vi "NextToken.vi"(7 "error in (no error)":errorcluster, 9 "Index In":i32, 10 "JSON String":string) -> (0 "error out":errorcluster, 1 "TOKEN":T1, 2 "Index Out":i32, 3 "JSON String Passthrough":string)   [LabVIEW 2010, in "i3-json.lvlib"]
doc: "Use this template to build a VI to use as a subVI."
uses:
  i3-json.lvlib
  Token.ctl
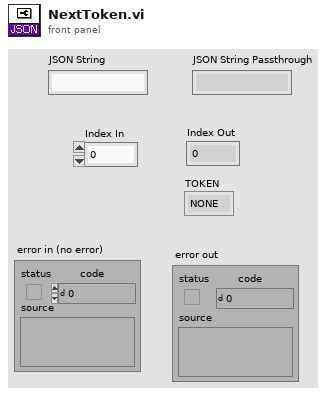
[diagram p1: front panel]
types:
  T1 = typedef "i3-json.lvlib/Token.ctl" = enum16{"NONE", "CURLY_OPEN", "CURLY_CLOSE", "SQUARED_OPEN", "SQUARED_CLOSE", "COLON", "COMMA", "STRING", "NUMBER", "TRUE", "FALSE", "NULL"}
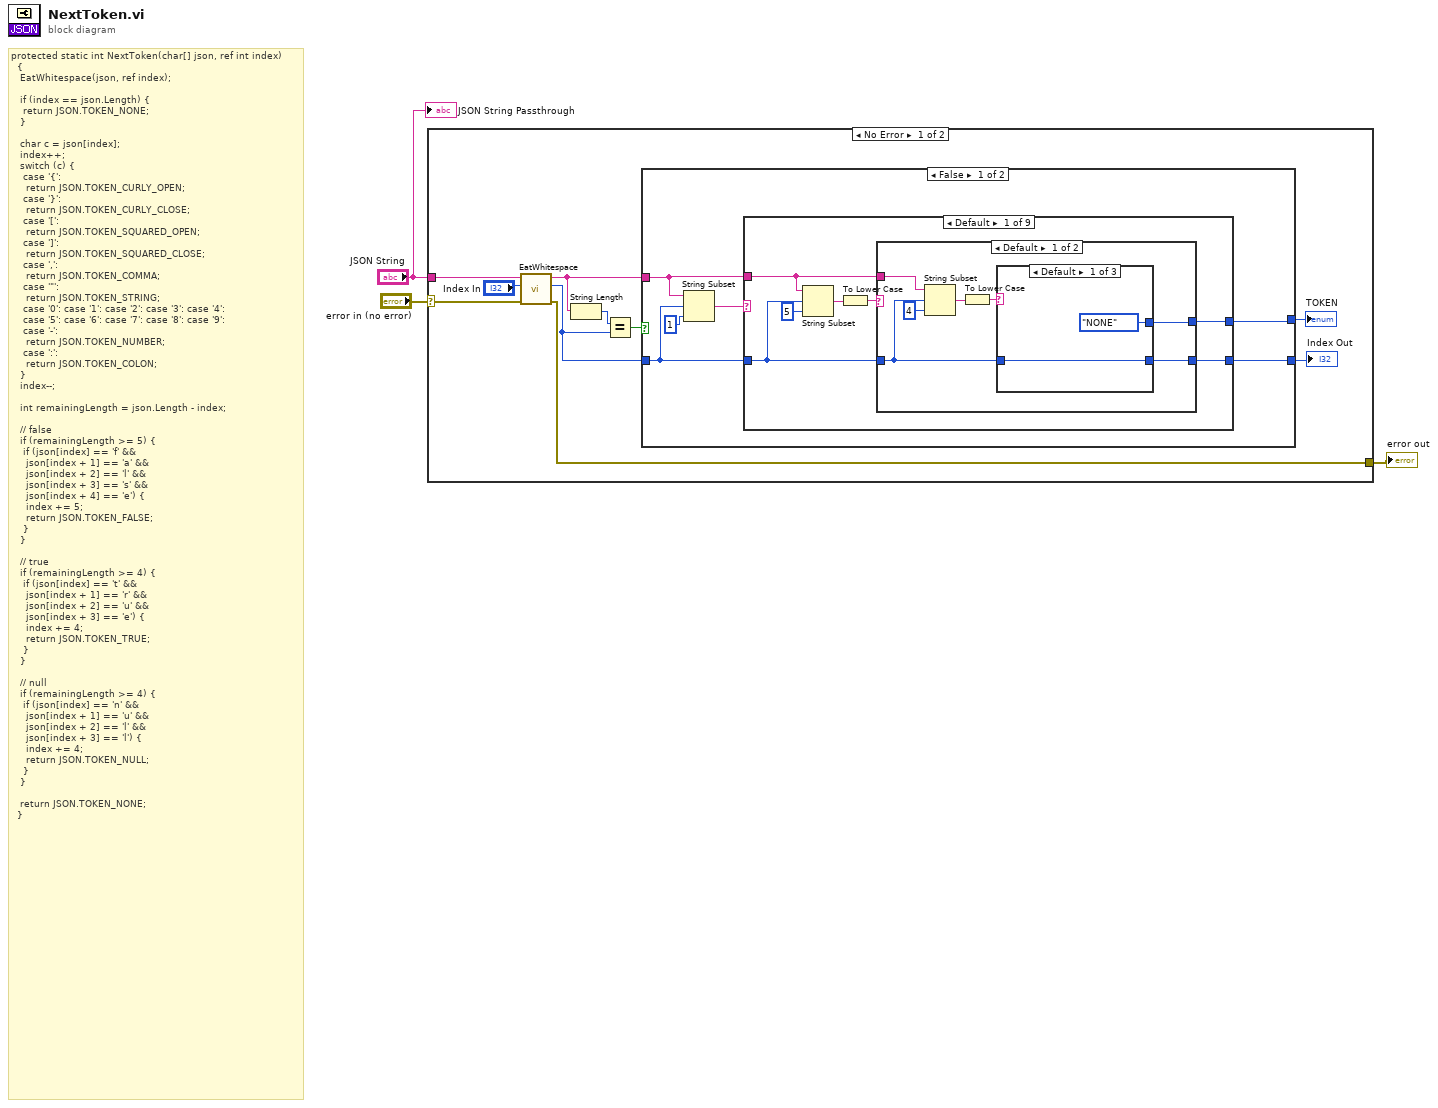
[diagram p0: block diagram]
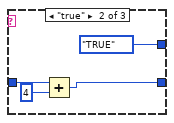
[diagram p2: hidden frame]
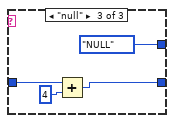
[diagram p3: hidden frame]
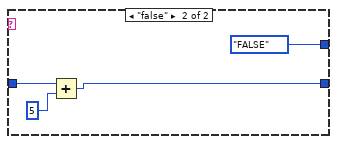
[diagram p4: hidden frame]
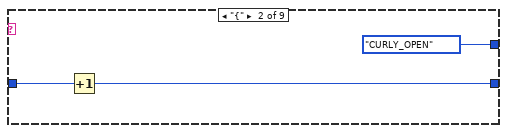
[diagram p5: hidden frame]
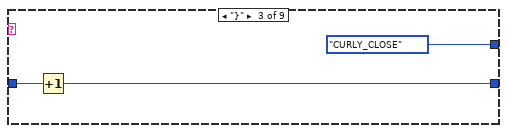
[diagram p6: hidden frame]
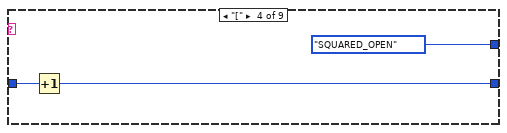
[diagram p7: hidden frame]
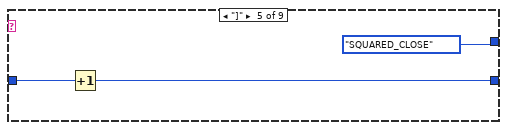
[diagram p8: hidden frame]
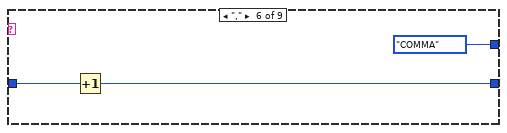
[diagram p9: hidden frame]
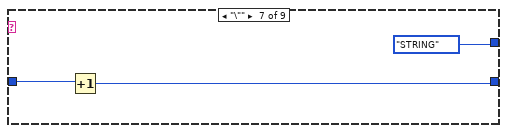
[diagram p10: hidden frame]
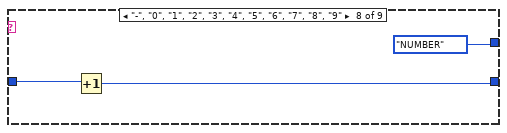
[diagram p11: hidden frame]
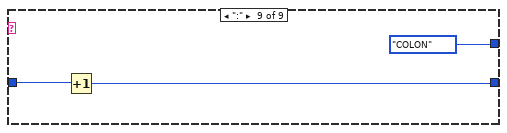
[diagram p12: hidden frame]
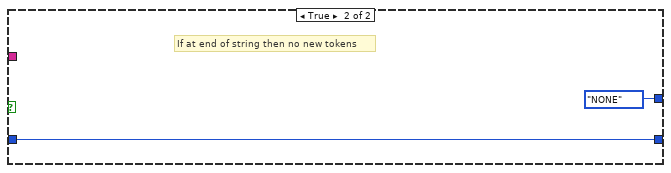
[diagram p13: hidden frame]
diagram:
  # "protected static int NextToken(char[] json, ref int index)\n\t\t{\n\t\t\tEatWhitespace(json, ref index);\n\n\t\t\tif (index == json.Length) {\n\t\t\t\treturn JSON.TOKEN_NONE;\n\t\t\t}\n\n\t\t\tchar c = json[index];\n\t\t\tindex++;\n\t\t\tswitch (c) {\n\t\t\t\tcase '{':\n\t\t\t\t\treturn JSON.TOKEN_CURLY_OPEN;\n\t\t\t\tcase '}':\n\t\t\t\t\treturn JSON.TOKEN_CURLY_CLOSE;\n\t\t\t\tcase '[':\n\t\t\t\t\treturn JSON.TOKEN_SQUARED_OPEN;\n\t\t\t\tcase ']':\n\t\t\t\t\treturn JSON.TOKEN_SQUARED_CLOSE;\n\t\t\t\tcase ',':\n\t\t\t\t\treturn JSON.TOKEN_COMMA;\n\t\t\t\tcase '\"':\n\t\t\t\t\treturn JSON.TOKEN_STRING;\n\t\t\t\tcase '0': case '1': case '2': case '3': case '4':\n\t\t\t\tcase '5': case '6': case '7': case '8': case '9':\n\t\t\t\tcase '-':\n\t\t\t\t\treturn JSON.TOKEN_NUMBER;\n\t\t\t\tcase ':':\n\t\t\t\t\treturn JSON.TOKEN_COLON;\n\t\t\t}\n\t\t\tindex--;\n\n\t\t\tint remainingLength = json.Length - index;\n\n\t\t\t// false\n\t\t\tif (remainingLength >= 5) {\n\t\t\t\tif (json[index] == 'f' &&\n\t\t\t\t\tjson[index + 1] == 'a' &&\n\t\t\t\t\tjson[index + 2] == 'l' &&\n\t\t\t\t\tjson[index + 3] == 's' &&\n\t\t\t\t\tjson[index + 4] == 'e') {\n\t\t\t\t\tindex += 5;\n\t\t\t\t\treturn JSON.TOKEN_FALSE;\n\t\t\t\t}\n\t\t\t}\n\n\t\t\t// true\n\t\t\tif (remainingLength >= 4) {\n\t\t\t\tif (json[index] == 't' &&\n\t\t\t\t\tjson[index + 1] == 'r' &&\n\t\t\t\t\tjson[index + 2] == 'u' &&\n\t\t\t\t\tjson[index + 3] == 'e') {\n\t\t\t\t\tindex += 4;\n\t\t\t\t\treturn JSON.TOKEN_TRUE;\n\t\t\t\t}\n\t\t\t}\n\n\t\t\t// null\n\t\t\tif (remainingLength >= 4) {\n\t\t\t\tif (json[index] == 'n' &&\n\t\t\t\t\tjson[index + 1] == 'u' &&\n\t\t\t\t\tjson[index + 2] == 'l' &&\n\t\t\t\t\tjson[index + 3] == 'l') {\n\t\t\t\t\tindex += 4;\n\t\t\t\t\treturn JSON.TOKEN_NULL;\n\t\t\t\t}\n\t\t\t}\n\n\t\t\treturn JSON.TOKEN_NONE;\n\t\t}"
  n1 = case shown="No Error" "error in (no error)" {
    selector: "error in (no error)" -> [w12 w74]
    tunnel: [w5 w74] -> w2
    tunnel: "JSON String" -> [w8 _]
    frame No Error {
      n2 = call "EatWhitespace.vi"("error in (no error)"=w12, "Index In"="Index In", "JSON String"=w8) -> ("error out"=w5:errorcluster, "Index Out"=w7:i32, "JSON String Passthrough"=w4:string)  [unwired: 6 in]
      n3 = String Length(string=w4) -> (length=w11:i32)
      n4 = Equal?(x=w11, y=w7) -> (x = y?=w10:bool)
      n5 = case shown="False" w10 {
        tunnel: [w15 Token."NONE" ("TOKEN")] -> w9
        tunnel: w7 -> [w17 w72]
        tunnel: w4 -> [w14 _]
        tunnel: [w16 w72] -> w6
        frame False {
          n6 = String Subset(string=w14, offset (0)=w17, length (rest)=1 ("length (rest)")) -> (substring=w18:string)
          n7 = case shown="Default" w18 {
            tunnel: w17 -> [w23 w50 w52 w55 w57 w61 w64 w67 w70]
            tunnel: [w22 w49 w51 w54 w58 w60 w63 w66 w69] -> w16
            tunnel: [w21 Token."CURLY_OPEN" ("TOKEN") Token."CURLY_CLOSE" ("TOKEN") Token."SQUARED_OPEN" ("TOKEN") Token."SQUARED_CLOSE" ("TOKEN") Token."COMMA" ("TOKEN") Token."STRING" ("TOKEN") Token."NUMBER" ("TOKEN") Token."COLON" ("TOKEN")] -> w15
            tunnel: w14 -> [w20 _ _ _ _ _ _ _ _]
            frame Default {
              n8 = String Subset(string=w20, offset (0)=w23, length (rest)=5 ("length (rest)")) -> (substring=w25:string)
              n9 = To Lower Case(string=w25) -> (all lower case string=w24:string)
              n10 = case shown="Default" w24 {
                tunnel: w23 -> [w29 w47]
                tunnel: [w28 w45] -> w22
                tunnel: [w27 Token."FALSE" ("TOKEN")] -> w21
                tunnel: w20 -> [w31 _]
                frame Default {
                  n11 = String Subset(string=w31, offset (0)=w29, length (rest)=4 ("length (rest)")) -> (substring=w33:string)
                  n12 = To Lower Case(string=w33) -> (all lower case string=w30:string)
                  n13 = case shown="Default" w30 {
                    tunnel: w29 -> [w35 w39 w43]
                    tunnel: [w35 w37 w41] -> w28
                    tunnel: [Token."NONE" ("TOKEN") Token."TRUE" ("TOKEN") Token."NULL" ("TOKEN")] -> w27
                    frame Default {
                    }
                    frame "true" {
                      n14 = Add(x=w39, y=4) -> (x+y=w37:i32)
                    }
                    frame "null" {
                      n15 = Add(x=w43, y=4) -> (x+y=w41:i32)
                    }
                  }
                }
                frame "false" {
                  n16 = Add(x=w47, y=5) -> (x+y=w45:i32)
                }
              }
            }
            frame "{" {
              n17 = Increment(x=w50) -> (x+1=w49:i32)
            }
            frame "}" {
              n18 = Increment(x=w52) -> (x+1=w51:i32)
            }
            frame "[" {
              n19 = Increment(x=w55) -> (x+1=w54:i32)
            }
            frame "]" {
              n20 = Increment(x=w57) -> (x+1=w58:i32)
            }
            frame "," {
              n21 = Increment(x=w61) -> (x+1=w60:i32)
            }
            frame "\"" {
              n22 = Increment(x=w64) -> (x+1=w63:i32)
            }
            frame "-", "0", "1", "2", "3", "4", "5", "6", "7", "8", "9" {
              n23 = Increment(x=w67) -> (x+1=w66:i32)
            }
            frame ":" {
              n24 = Increment(x=w70) -> (x+1=w69:i32)
            }
          }
        }
        frame True {
          # "If at end of string then no new tokens"
        }
      }
      "Index Out" <- w6
      "TOKEN" <- w9
    }
    frame Error {
    }
  }
  "error out" <- w2
  "JSON String Passthrough" <- "JSON String"
